vi "HF2LI_Manage_Monitor.vi"(8 "Global Status (in)":T1={"X 1 (Vrms)"=2.7056741238785867e-06, "Y 1 (Vrms)"=-1.312399113553479e-06, "A 1 (Vpk)"=0.39999694821890425, "A 2 (Vpk)"=0.04999580380099335, "Output 1"=FALSE, "Output 2"=FALSE, "f 1 (Hz)"=201.99999966052928, "f 2 (Hz)"=201.99999966052928, "X 2 (Vrms)"=3.017847906110667e-06, "Y 2 (Vrms)"=-2.261753825762805e-06, "Output 1 Add"=FALSE, "Output 2 Add"=FALSE, "Input Min %"=0.0, "Input Max %"=0.0}, 11 "System Monitor Variables (in)":T2) -> (0 "Monitor out":T1={"X 1 (Vrms)"=2.7056741238785867e-06, "Y 1 (Vrms)"=-1.312399113553479e-06, "A 1 (Vpk)"=0.39999694821890425, "A 2 (Vpk)"=0.04999580380099335, "Output 1"=FALSE, "Output 2"=FALSE, "f 1 (Hz)"=201.99999966052928, "f 2 (Hz)"=201.99999966052928, "X 2 (Vrms)"=3.017847906110667e-06, "Y 2 (Vrms)"=-2.261753825762805e-06, "Output 1 Add"=FALSE, "Output 2 Add"=FALSE, "Input Min %"=0.0, "Input Max %"=0.0}, 3 "System Monitor Variables (out)":T2)   [LabVIEW 2019]
uses:
  Global/Global Variables/System Monitor Cluster.ctl
  HF2LI/HF2LI.ctl
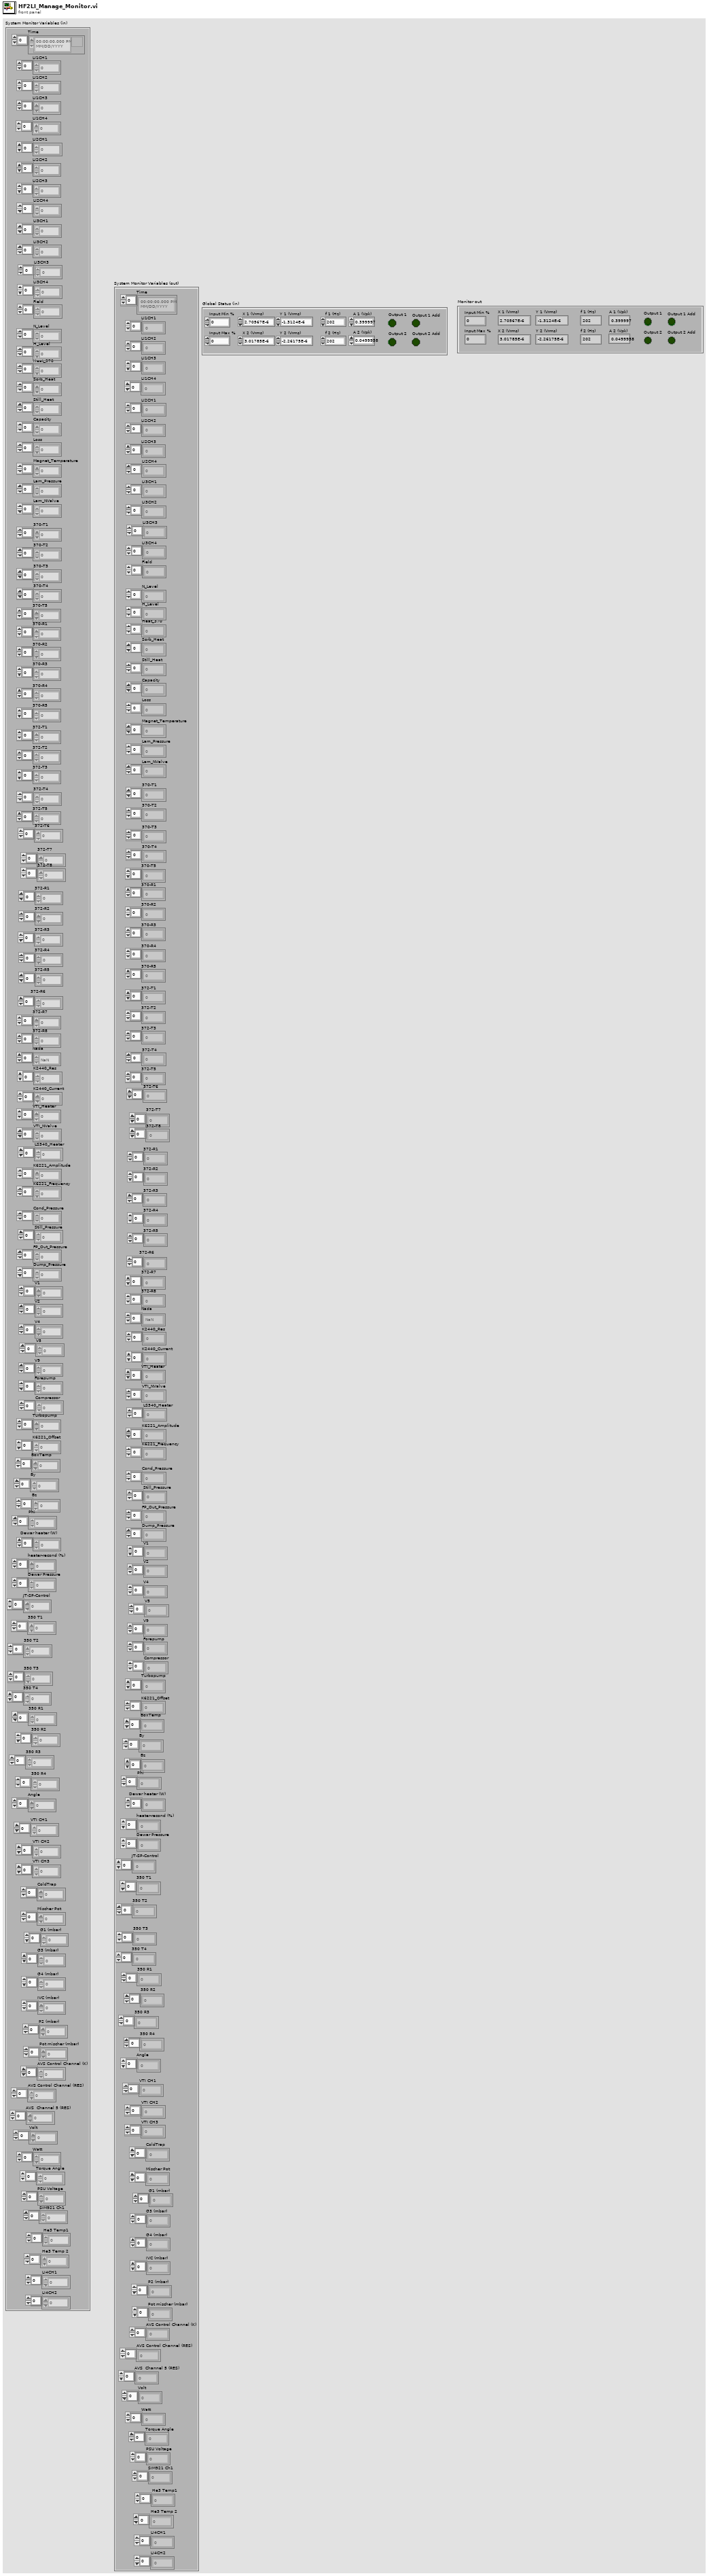
[diagram p1: front panel]
types:
  T1 = typedef "HF2LI.ctl" = cluster{"X 1 (Vrms)":dbl, "Y 1 (Vrms)":dbl, "A 1 (Vpk)":dbl, "A 2 (Vpk)":dbl, "Output 1":bool, "Output 2":bool, "f 1 (Hz)":dbl, "f 2 (Hz)":dbl, "X 2 (Vrms)":dbl, "Y 2 (Vrms)":dbl, "Output 1 Add":bool, "Output 2 Add":bool, "Input Min %":dbl, "Input Max %":dbl}
  T2 = typedef "System Monitor Cluster.ctl" = cluster{"Time":timestamp[], "LI1CH1":dbl[], "LI1CH2":dbl[], "LI2CH1":dbl[], "LI2CH2":dbl[], "LI3CH1":dbl[], "LI3CH2":dbl[], "Field":dbl[], "N_Level":dbl[], "H_Level":dbl[], "Heat_370":dbl[], "Sorb_Heat":dbl[], "Still_Heat":dbl[], "Capacity":dbl[], "Loss":dbl[], "Magnet_Temperature":dbl[], "Lam_Pressure":dbl[], "Lam_NValve":dbl[], "370-T1":dbl[], "370-T2":dbl[], "370-T3":dbl[], "370-T4":dbl[], "370-T5":dbl[], "370-R1":dbl[], "370-R2":dbl[], "370-R3":dbl[], "370-R4":dbl[], "370-R5":dbl[], "372-T1":dbl[], "372-T2":dbl[], "372-T3":dbl[], "372-T4":dbl[], "372-T5":dbl[], "372-T6":dbl[], "372-R1":dbl[], "372-R2":dbl[], "372-R3":dbl[], "372-R4":dbl[], "372-R5":dbl[], "372-R6":dbl[], "Nada":dbl[], "K2440_Res":dbl[], "K2440_Current":dbl[], "VTI_Heater":dbl[], "VTI_NValve":dbl[], "LS340_Heater":dbl[], "K6221_Amplitude":dbl[], "K6221_Frequency":dbl[], "Cond_Pressure":dbl[], "Still_Pressure":dbl[], "FP_Out_Pressure":dbl[], "Dump_Pressure":dbl[], "V1":dbl[], "V2":dbl[], "V4":dbl[], "V5":dbl[], "V9":dbl[], "Forepump":dbl[], "Compressor":dbl[], "K6221_Offset":dbl[], "BoxTemp":dbl[], "By":dbl[], "Bz":dbl[], "Phi":dbl[], "heater-recond (%)":dbl[], "Dewar Pressure ":dbl[], "JT-SP-Control":dbl[], "350 T1":dbl[], "350 T2":dbl[], "350 T3":dbl[], "350 T4":dbl[], "350 R1":dbl[], "350 R2":dbl[], "350 R3":dbl[], "350 R4":dbl[], "Angle":dbl[], "VTI CH1":dbl[], "VTI CH2":dbl[], "VTI CH3":dbl[], "ColdTrap":dbl[], "Mischer Pot":dbl[], "G1 (mbar)":dbl[], "G3 (mbar) ":dbl[], "G4 (mbar)":dbl[], "IVC (mbar)":dbl[], "P2 (mbar) ":dbl[], "Pot mischer (mbar)":dbl[], "AVS Control Channel (K)":dbl[], "AVS Control Channel (RES)":dbl[], "AVS  Channel 5 (RES) ":dbl[], "LI3CH3":dbl[], "LI3CH4":dbl[], "LI1CH3":dbl[], "LI1CH4":dbl[], "LI2CH3":dbl[], "LI2CH4":dbl[], "Volt":dbl[], "Watt":dbl[], "Torque Angle":dbl[], "Dewar heater (W)":dbl[], "PSU Voltage":dbl[], "Turbopump":dbl[], "372-R7":dbl[], "372-T7":dbl[], "SIM921 Ch1":dbl[], " He3 Temp1":dbl[], " He3 Temp 2":dbl[], "LI4CH1":dbl[], "LI4CH2":dbl[], "372-T8":dbl[], "372-R8":dbl[]}
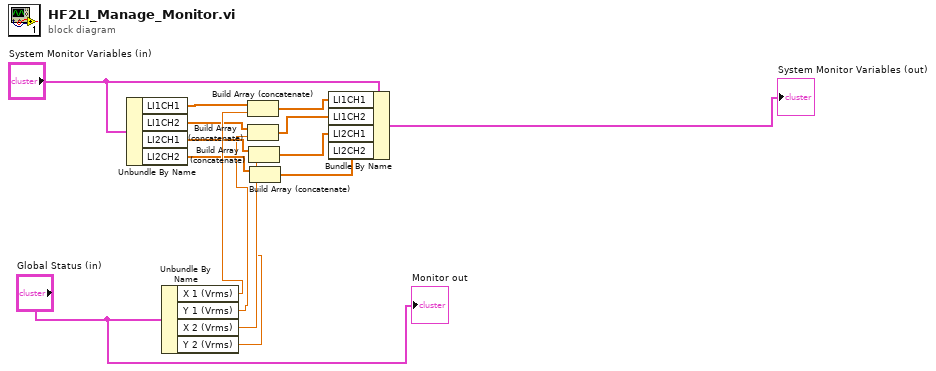
[diagram p0: block diagram]
diagram:
  n1 = Unbundle By Name("System Monitor Variables (in)") -> ("LI1CH1"=w13:dbl[], "LI1CH2"=w5:dbl[], "LI2CH1"=w6:dbl[], "LI2CH2"=w7:dbl[])
  n2 = Unbundle By Name("Global Status (in)") -> ("X 1 (Vrms)"=w11:dbl, "Y 1 (Vrms)"=w4:dbl, "X 2 (Vrms)"=w3:dbl, "Y 2 (Vrms)"=w2:dbl)
  n3 = Build Array (concatenate)(w13, w11) -> (w12:dbl[])
  n4 = Build Array (concatenate)(w5, w4) -> (w10:dbl[])
  n5 = Build Array (concatenate)(w6, w3) -> (w9:dbl[])
  n6 = Build Array (concatenate)(w7, w2) -> (w8:dbl[])
  n7 = Bundle By Name(cluster="System Monitor Variables (in)", "LI1CH1"=w12, "LI1CH2"=w10, "LI2CH1"=w9, "LI2CH2"=w8) -> (→"System Monitor Variables (out)":T2)
  "Monitor out" <- "Global Status (in)"
